vi "Peak Detector (multiple).vi"(6 "Width Unit (points)":enum16{"Points", "Data"}(ring), 8 "error in (no error)":errorcluster, 9 "width":dbl=3.0 min=3.0, 10 "threshold":dbl format="%0.2f", 11 "XY-data":cluster{"X-array":dbl[], "Y-array":dbl[]}[](array[cluster])) -> (0 "error out":errorcluster, 1 "Amplitudes":cluster{"Amplitudes":dbl[]}[](array[cluster]), 2 "Locations":cluster{"Locations":dbl[]}[](array[cluster]), 3 "XY-data out":cluster{"X-array":dbl[], "Y-array":dbl[]}[](array[cluster]) {"Y-array" format="%.2p"; "X-array" format="%.2p"})   [LabVIEW 2019, in "xy_utilities.lvlib"]
doc: "Find <b>peaks</b> in <b>XY-data</b>'s Y-Array.\n\nWire data to the data input to determine the polymorphic instance to use or manually select the instance."
uses:
  xy_utilities.lvlib
  Private/X Units.vi
  Private/X Array Range to Index.vi
  <vilib>/Analysis/8numeric.llb/Peak Detector.vi
  <userlib>/_MGI/1D Array/MGI Interpolate 1D Array Extended.vi
  <vilib>/Utility/error.llb/Error Cluster From Error Code.vi
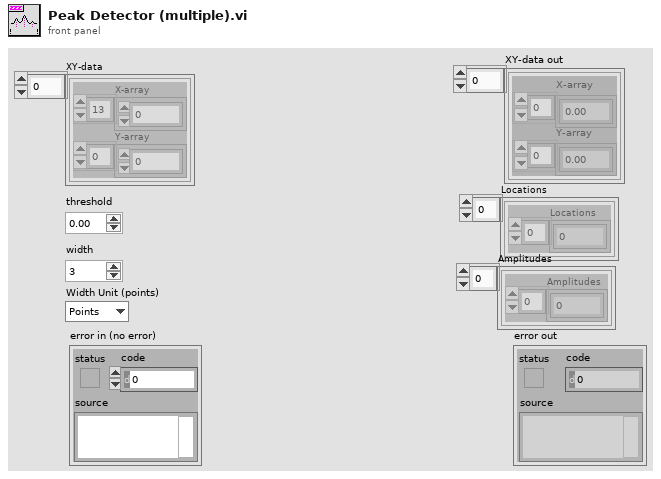
[diagram p1: front panel]
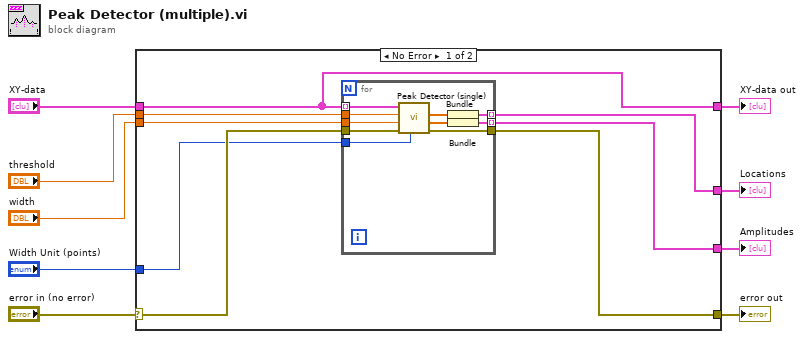
[diagram p0: block diagram]
diagram:
  n1 = case shown="No Error" "error in (no error)" {
    selector: "error in (no error)" -> [w17 w29]
    tunnel: [w16 w29] -> w8
    tunnel: "XY-data" -> [w10 w28]
    tunnel: [w10 w28] -> w6
    tunnel: "width" -> [w15 _]
    tunnel: "threshold" -> [w14 _]
    tunnel: [w13 _] -> w3
    tunnel: [w12 _] -> w2
    tunnel: "Width Unit (points)" -> [w11 _]
    frame No Error {
      n2 = for {
        tunnel: w10 -> [w27] mode=indexing
        tunnel: w17 -> [w26]
        tunnel: [w25] -> w16
        tunnel: w15 -> [w24]
        tunnel: w14 -> [w23]
        tunnel: [w20] -> w13 mode=indexing
        tunnel: [w19] -> w12 mode=indexing
        tunnel: w11 -> [w18]
        n3 = call "Peak Detector (single).vi"("Width Unit (points)"=w18, "error in (no error)"=w26, "width"=w24, "threshold"=w23, "XY-data"=w27) -> ("error out"=w25:errorcluster, "Amplitudes"=w21:dbl[], "Locations"=w22:dbl[])  [unwired: 3 in, 1 out]
        n4 = Bundle("Locations"=w22) -> (w20:cluster{"Locations":dbl[]})  [unwired: 1 in]
        n5 = Bundle("Amplitudes"=w21) -> (w19:cluster{"Amplitudes":dbl[]})  [unwired: 1 in]
      }
    }
    frame Error {
    }
  }
  "error out" <- w8
  "XY-data out" <- w6
  "Locations" <- w3
  "Amplitudes" <- w2
